vi "LoopConfigStopCond.vi"(8 "Error":errorcluster[](array[cluster]), 10 "StopCondition":variant, 11 "Test.lvclass":refnum<class "Test.lvclass">) -> (0 "Error":errorcluster[](array[cluster]), 3 "Test.lvclass":refnum<class "Test.lvclass">)   [LabVIEW 2014, in "Test.lvclass"]
uses:
  Test.lvclass
  Typedef/LoopStopCondition.ctl
  Test.lvclass/Test.ctl
  Accessors/Write LoopStopCondition.vi
  Accessors/Read ErrorSeverity.vi
  <userlib>/NIST/NISTErrorLib/NISTErrorLib.lvlib
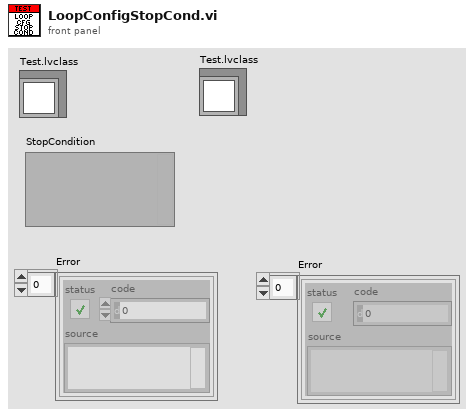
[diagram p1: front panel]
types:
  T1 = typedef "Test.lvclass/LoopStopCondition.ctl" = cluster{"Name":string, "StopCondition":variant}
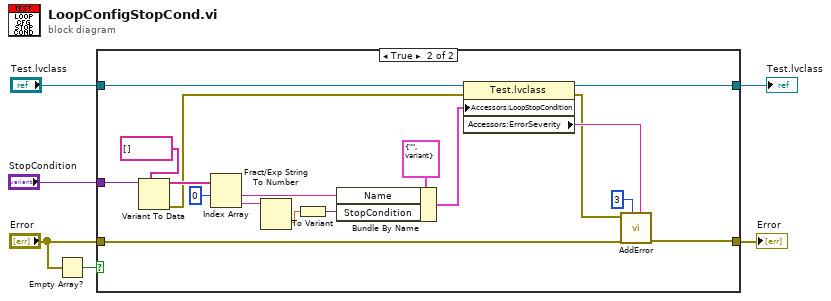
[diagram p0: block diagram]
diagram:
  n1 = Empty Array?(array="Error") -> (empty?=w5:bool)
  n2 = case shown="True" w5 {
    tunnel: "Error" -> [w8 w14]
    tunnel: [w8 w9] -> w1
    tunnel: "Test.lvclass" -> [w7 w21]
    tunnel: [w7 w15] -> w3
    tunnel: "StopCondition" -> [_ w26]
    frame False {
    }
    frame True {
      n3 = Variant To Data(type=string[] [], Variant=w26) -> (data=w24:string[], error out=w13:errorcluster)  [unwired: 1 in]
      n4 = Index Array(array=w24, index #1=0 ("index")) -> (element #1=w19:string, element #2=w22:string)  [unwired: 1 in]
      n5 = Fract/Exp String To Number(string=w22) -> (number=w18:dbl)  [unwired: 3 in, 1 out]
      n6 = To Variant(anything=w18) -> (Variant=w17:variant)
      n7 = Bundle By Name(cluster=T1 {"Name"="", "StopCondition"=variant} ("LoopStopCondition"), "Name"=w19, "StopCondition"=w17) -> (w16:T1)
      n8 = property class="Test.lvclass"(reference=w21, error in=w13, "Accessors:LoopStopCondition"=w16) -> (reference out=w15:refnum<class "Test.lvclass">, error out=w10:errorcluster, "Accessors:ErrorSeverity"=w12:string)
      n9 = call <userlib>:"AddError.vi"("Severity"=w12, "Priority"=u8 3, "ErrorArray"=w14, "error in (no error)"=w10) -> ("ErrorArray"=w9:errorcluster[])  [unwired: 6 in, 1 out]
    }
  }
  "Test.lvclass" <- w3
  "Error" <- w1
